vi "Frame Data Message Create.vi"(8 "error in (no error)":errorcluster, 10 "Video Frame":refnum<class "Video Frame.lvclass">, 11 "Frame Data Message in":refnum<class "Frame Data Message.lvclass">) -> (0 "error out":errorcluster, 3 "Frame Data Message out":refnum<class "Frame Data Message.lvclass">)   [LabVIEW 2018, in "Frame Data Message.lvclass"]
uses:
  Frame Data Message.lvclass
  Video Frame/Video Frame.lvclass
  Frame Data Message.lvclass/Frame Data Message.ctl
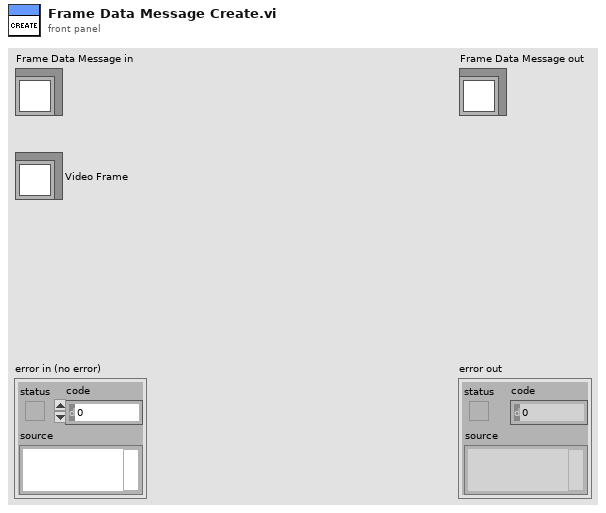
[diagram p1: front panel]
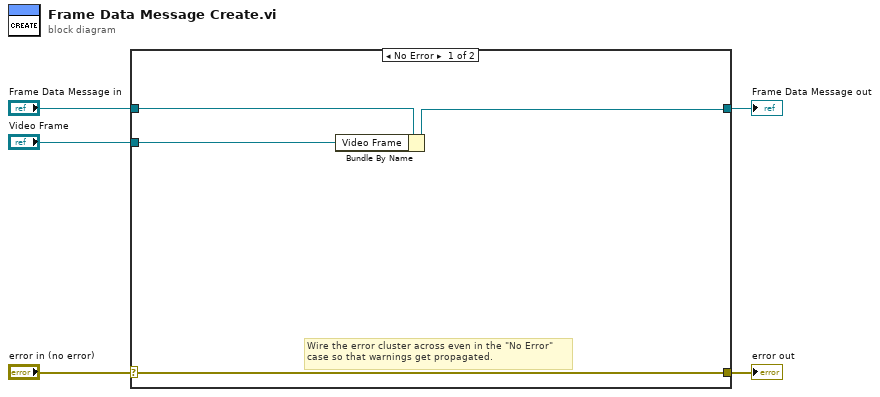
[diagram p0: block diagram]
diagram:
  n1 = case shown="No Error" "error in (no error)" {
    selector: "error in (no error)" -> [w9 w11]
    tunnel: [w9 w11] -> w4
    tunnel: [w6 w10] -> w2
    tunnel: "Frame Data Message in" -> [w8 w10]
    tunnel: "Video Frame" -> [w7 _]
    frame No Error {
      # "Wire the error cluster across even in the \"No Error\"\ncase so that warnings get propagated."
      n2 = Bundle By Name(cluster=w8, "Video Frame"=w7) -> (w6:refnum<class "Frame Data Message.lvclass">)
    }
    frame Error {
    }
  }
  "error out" <- w4
  "Frame Data Message out" <- w2
